vi "初始化.vi"(3 "Container State":T8 caption="容器状态", 4 "Previous State":variant caption="前期状态", 5 "Previous Version":T7 caption="前期版本") -> (2 "Current State":T1 caption="当前状态" {"配置信息"."间隔启动"."启动命令" items=["", "水样测试", "标样核查", "零点核查", "跨度核查", "空白测试", "平行样测试", "加标回收", "空白校准", "标样校准"]; "配置信息"."定点周期"."启动命令 24" items=["", "水样测试", "标样核查", "零点核查", "跨度核查", "空白测试", "平行样测试", "加标回收", "空白校准", "标样校准"]; "配置信息"."定点周期"."启动命令 23" items=["", "水样测试", "标样核查", "零点核查", "跨度核查", "空白测试", "平行样测试", "加标回收", "空白校准", "标样校准"]; "配置信息"."定点周期"."启动命令 22" items=["", "水样测试", "标样核查", "零点核查", "跨度核查", "空白测试", "平行样测试", "加标回收", "空白校准", "标样校准"]; "配置信息"."定点周期"."启动命令 21" items=["", "水样测试", "标样核查", "零点核查", "跨度核查", "空白测试", "平行样测试", "加标回收", "空白校准", "标样校准"]; "配置信息"."定点周期"."启动命令 20" items=["", "水样测试", "标样核查", "零点核查", "跨度核查", "空白测试", "平行样测试", "加标回收", "空白校准", "标样校准"]; "配置信息"."定点周期"."启动命令 19" items=["", "水样测试", "标样核查", "零点核查", "跨度核查", "空白测试", "平行样测试", "加标回收", "空白校准", "标样校准"]; "配置信息"."定点周期"."启动命令 18" items=["", "水样测试", "标样核查", "零点核查", "跨度核查", "空白测试", "平行样测试", "加标回收", "空白校准", "标样校准"]; "配置信息"."定点周期"."启动命令 17" items=["", "水样测试", "标样核查", "零点核查", "跨度核查", "空白测试", "平行样测试", "加标回收", "空白校准", "标样校准"]; "配置信息"."定点周期"."启动命令 16" items=["", "水样测试", "标样核查", "零点核查", "跨度核查", "空白测试", "平行样测试", "加标回收", "空白校准", "标样校准"]; "配置信息"."定点周期"."启动命令 15" items=["", "水样测试", "标样核查", "零点核查", "跨度核查", "空白测试", "平行样测试", "加标回收", "空白校准", "标样校准"]; "配置信息"."定点周期"."启动命令 14" items=["", "水样测试", "标样核查", "零点核查", "跨度核查", "空白测试", "平行样测试", "加标回收", "空白校准", "标样校准"]; "配置信息"."定点周期"."启动命令 13" items=["", "水样测试", "标样核查", "零点核查", "跨度核查", "空白测试", "平行样测试", "加标回收", "空白校准", "标样校准"]; "配置信息"."定点周期"."启动命令 12" items=["", "水样测试", "标样核查", "零点核查", "跨度核查", "空白测试", "平行样测试", "加标回收", "空白校准", "标样校准"]; "配置信息"."定点周期"."启动命令 11" items=["", "水样测试", "标样核查", "零点核查", "跨度核查", "空白测试", "平行样测试", "加标回收", "空白校准", "标样校准"]; "配置信息"."定点周期"."启动命令 10" items=["", "水样测试", "标样核查", "零点核查", "跨度核查", "空白测试", "平行样测试", "加标回收", "空白校准", "标样校准"]; "配置信息"."定点周期"."启动命令 9" items=["", "水样测试", "标样核查", "零点核查", "跨度核查", "空白测试", "平行样测试", "加标回收", "空白校准", "标样校准"]; "配置信息"."定点周期"."启动命令 8" items=["", "水样测试", "标样核查", "零点核查", "跨度核查", "空白测试", "平行样测试", "加标回收", "空白校准", "标样校准"]; "配置信息"."定点周期"."启动命令 7" items=["", "水样测试", "标样核查", "零点核查", "跨度核查", "空白测试", "平行样测试", "加标回收", "空白校准", "标样校准"]; "配置信息"."定点周期"."启动命令 6" items=["", "水样测试", "标样核查", "零点核查", "跨度核查", "空白测试", "平行样测试", "加标回收", "空白校准", "标样校准"]; "配置信息"."定点周期"."启动命令 5" items=["", "水样测试", "标样核查", "零点核查", "跨度核查", "空白测试", "平行样测试", "加标回收", "空白校准", "标样校准"]; "配置信息"."定点周期"."启动命令 4" items=["", "水样测试", "标样核查", "零点核查", "跨度核查", "空白测试", "平行样测试", "加标回收", "空白校准", "标样校准"]; "配置信息"."定点周期"."启动命令 3" items=["", "水样测试", "标样核查", "零点核查", "跨度核查", "空白测试", "平行样测试", "加标回收", "空白校准", "标样校准"]; "配置信息"."定点周期"."启动命令 2" items=["", "水样测试", "标样核查", "零点核查", "跨度核查", "空白测试", "平行样测试", "加标回收", "空白校准", "标样校准"]; "配置信息"."定点周期"."启动命令" items=["", "水样测试", "标样核查", "零点核查", "跨度核查", "空白测试", "平行样测试", "加标回收", "空白校准", "标样校准"]})   [LabVIEW 2016, in "定时设置.xctl"]
uses:
  <vilib>/_xctls/Container State.ctl
  <vilib>/_xctls/Version.ctl
  <vilib>/_xctls/XControlSupport.lvlib
panel:
  in  "Default Indicator State":T1 caption="默认显示控件状态" {"配置信息"."间隔启动"."启动命令" items=["", "水样测试", "标样核查", "零点核查", "跨度核查", "空白测试", "平行样测试", "加标回收", "空白校准", "标样校准"]; "配置信息"."定点周期"."启动命令 24" items=["", "水样测试", "标样核查", "零点核查", "跨度核查", "空白测试", "平行样测试", "加标回收", "空白校准", "标样校准"]; "配置信息"."定点周期"."启动命令 23" items=["", "水样测试", "标样核查", "零点核查", "跨度核查", "空白测试", "平行样测试", "加标回收", "空白校准", "标样校准"]; "配置信息"."定点周期"."启动命令 22" items=["", "水样测试", "标样核查", "零点核查", "跨度核查", "空白测试", "平行样测试", "加标回收", "空白校准", "标样校准"]; "配置信息"."定点周期"."启动命令 21" items=["", "水样测试", "标样核查", "零点核查", "跨度核查", "空白测试", "平行样测试", "加标回收", "空白校准", "标样校准"]; "配置信息"."定点周期"."启动命令 20" items=["", "水样测试", "标样核查", "零点核查", "跨度核查", "空白测试", "平行样测试", "加标回收", "空白校准", "标样校准"]; "配置信息"."定点周期"."启动命令 19" items=["", "水样测试", "标样核查", "零点核查", "跨度核查", "空白测试", "平行样测试", "加标回收", "空白校准", "标样校准"]; "配置信息"."定点周期"."启动命令 18" items=["", "水样测试", "标样核查", "零点核查", "跨度核查", "空白测试", "平行样测试", "加标回收", "空白校准", "标样校准"]; "配置信息"."定点周期"."启动命令 17" items=["", "水样测试", "标样核查", "零点核查", "跨度核查", "空白测试", "平行样测试", "加标回收", "空白校准", "标样校准"]; "配置信息"."定点周期"."启动命令 16" items=["", "水样测试", "标样核查", "零点核查", "跨度核查", "空白测试", "平行样测试", "加标回收", "空白校准", "标样校准"]; "配置信息"."定点周期"."启动命令 15" items=["", "水样测试", "标样核查", "零点核查", "跨度核查", "空白测试", "平行样测试", "加标回收", "空白校准", "标样校准"]; "配置信息"."定点周期"."启动命令 14" items=["", "水样测试", "标样核查", "零点核查", "跨度核查", "空白测试", "平行样测试", "加标回收", "空白校准", "标样校准"]; "配置信息"."定点周期"."启动命令 13" items=["", "水样测试", "标样核查", "零点核查", "跨度核查", "空白测试", "平行样测试", "加标回收", "空白校准", "标样校准"]; "配置信息"."定点周期"."启动命令 12" items=["", "水样测试", "标样核查", "零点核查", "跨度核查", "空白测试", "平行样测试", "加标回收", "空白校准", "标样校准"]; "配置信息"."定点周期"."启动命令 11" items=["", "水样测试", "标样核查", "零点核查", "跨度核查", "空白测试", "平行样测试", "加标回收", "空白校准", "标样校准"]; "配置信息"."定点周期"."启动命令 10" items=["", "水样测试", "标样核查", "零点核查", "跨度核查", "空白测试", "平行样测试", "加标回收", "空白校准", "标样校准"]; "配置信息"."定点周期"."启动命令 9" items=["", "水样测试", "标样核查", "零点核查", "跨度核查", "空白测试", "平行样测试", "加标回收", "空白校准", "标样校准"]; "配置信息"."定点周期"."启动命令 8" items=["", "水样测试", "标样核查", "零点核查", "跨度核查", "空白测试", "平行样测试", "加标回收", "空白校准", "标样校准"]; "配置信息"."定点周期"."启动命令 7" items=["", "水样测试", "标样核查", "零点核查", "跨度核查", "空白测试", "平行样测试", "加标回收", "空白校准", "标样校准"]; "配置信息"."定点周期"."启动命令 6" items=["", "水样测试", "标样核查", "零点核查", "跨度核查", "空白测试", "平行样测试", "加标回收", "空白校准", "标样校准"]; "配置信息"."定点周期"."启动命令 5" items=["", "水样测试", "标样核查", "零点核查", "跨度核查", "空白测试", "平行样测试", "加标回收", "空白校准", "标样校准"]; "配置信息"."定点周期"."启动命令 4" items=["", "水样测试", "标样核查", "零点核查", "跨度核查", "空白测试", "平行样测试", "加标回收", "空白校准", "标样校准"]; "配置信息"."定点周期"."启动命令 3" items=["", "水样测试", "标样核查", "零点核查", "跨度核查", "空白测试", "平行样测试", "加标回收", "空白校准", "标样校准"]; "配置信息"."定点周期"."启动命令 2" items=["", "水样测试", "标样核查", "零点核查", "跨度核查", "空白测试", "平行样测试", "加标回收", "空白校准", "标样校准"]; "配置信息"."定点周期"."启动命令" items=["", "水样测试", "标样核查", "零点核查", "跨度核查", "空白测试", "平行样测试", "加标回收", "空白校准", "标样校准"]}
  in  "Default Control State":T1 caption="默认输入控件状态" {"配置信息"."间隔启动"."启动命令" items=["", "水样测试", "标样核查", "零点核查", "跨度核查", "空白测试", "平行样测试", "加标回收", "空白校准", "标样校准"]; "配置信息"."定点周期"."启动命令 24" items=["", "水样测试", "标样核查", "零点核查", "跨度核查", "空白测试", "平行样测试", "加标回收", "空白校准", "标样校准"]; "配置信息"."定点周期"."启动命令 23" items=["", "水样测试", "标样核查", "零点核查", "跨度核查", "空白测试", "平行样测试", "加标回收", "空白校准", "标样校准"]; "配置信息"."定点周期"."启动命令 22" items=["", "水样测试", "标样核查", "零点核查", "跨度核查", "空白测试", "平行样测试", "加标回收", "空白校准", "标样校准"]; "配置信息"."定点周期"."启动命令 21" items=["", "水样测试", "标样核查", "零点核查", "跨度核查", "空白测试", "平行样测试", "加标回收", "空白校准", "标样校准"]; "配置信息"."定点周期"."启动命令 20" items=["", "水样测试", "标样核查", "零点核查", "跨度核查", "空白测试", "平行样测试", "加标回收", "空白校准", "标样校准"]; "配置信息"."定点周期"."启动命令 19" items=["", "水样测试", "标样核查", "零点核查", "跨度核查", "空白测试", "平行样测试", "加标回收", "空白校准", "标样校准"]; "配置信息"."定点周期"."启动命令 18" items=["", "水样测试", "标样核查", "零点核查", "跨度核查", "空白测试", "平行样测试", "加标回收", "空白校准", "标样校准"]; "配置信息"."定点周期"."启动命令 17" items=["", "水样测试", "标样核查", "零点核查", "跨度核查", "空白测试", "平行样测试", "加标回收", "空白校准", "标样校准"]; "配置信息"."定点周期"."启动命令 16" items=["", "水样测试", "标样核查", "零点核查", "跨度核查", "空白测试", "平行样测试", "加标回收", "空白校准", "标样校准"]; "配置信息"."定点周期"."启动命令 15" items=["", "水样测试", "标样核查", "零点核查", "跨度核查", "空白测试", "平行样测试", "加标回收", "空白校准", "标样校准"]; "配置信息"."定点周期"."启动命令 14" items=["", "水样测试", "标样核查", "零点核查", "跨度核查", "空白测试", "平行样测试", "加标回收", "空白校准", "标样校准"]; "配置信息"."定点周期"."启动命令 13" items=["", "水样测试", "标样核查", "零点核查", "跨度核查", "空白测试", "平行样测试", "加标回收", "空白校准", "标样校准"]; "配置信息"."定点周期"."启动命令 12" items=["", "水样测试", "标样核查", "零点核查", "跨度核查", "空白测试", "平行样测试", "加标回收", "空白校准", "标样校准"]; "配置信息"."定点周期"."启动命令 11" items=["", "水样测试", "标样核查", "零点核查", "跨度核查", "空白测试", "平行样测试", "加标回收", "空白校准", "标样校准"]; "配置信息"."定点周期"."启动命令 10" items=["", "水样测试", "标样核查", "零点核查", "跨度核查", "空白测试", "平行样测试", "加标回收", "空白校准", "标样校准"]; "配置信息"."定点周期"."启动命令 9" items=["", "水样测试", "标样核查", "零点核查", "跨度核查", "空白测试", "平行样测试", "加标回收", "空白校准", "标样校准"]; "配置信息"."定点周期"."启动命令 8" items=["", "水样测试", "标样核查", "零点核查", "跨度核查", "空白测试", "平行样测试", "加标回收", "空白校准", "标样校准"]; "配置信息"."定点周期"."启动命令 7" items=["", "水样测试", "标样核查", "零点核查", "跨度核查", "空白测试", "平行样测试", "加标回收", "空白校准", "标样校准"]; "配置信息"."定点周期"."启动命令 6" items=["", "水样测试", "标样核查", "零点核查", "跨度核查", "空白测试", "平行样测试", "加标回收", "空白校准", "标样校准"]; "配置信息"."定点周期"."启动命令 5" items=["", "水样测试", "标样核查", "零点核查", "跨度核查", "空白测试", "平行样测试", "加标回收", "空白校准", "标样校准"]; "配置信息"."定点周期"."启动命令 4" items=["", "水样测试", "标样核查", "零点核查", "跨度核查", "空白测试", "平行样测试", "加标回收", "空白校准", "标样校准"]; "配置信息"."定点周期"."启动命令 3" items=["", "水样测试", "标样核查", "零点核查", "跨度核查", "空白测试", "平行样测试", "加标回收", "空白校准", "标样校准"]; "配置信息"."定点周期"."启动命令 2" items=["", "水样测试", "标样核查", "零点核查", "跨度核查", "空白测试", "平行样测试", "加标回收", "空白校准", "标样校准"]; "配置信息"."定点周期"."启动命令" items=["", "水样测试", "标样核查", "零点核查", "跨度核查", "空白测试", "平行样测试", "加标回收", "空白校准", "标样校准"]}
  # "分钟"
  # "次"
  # "分钟"
  # "次"
  # "分钟"
  # "次"
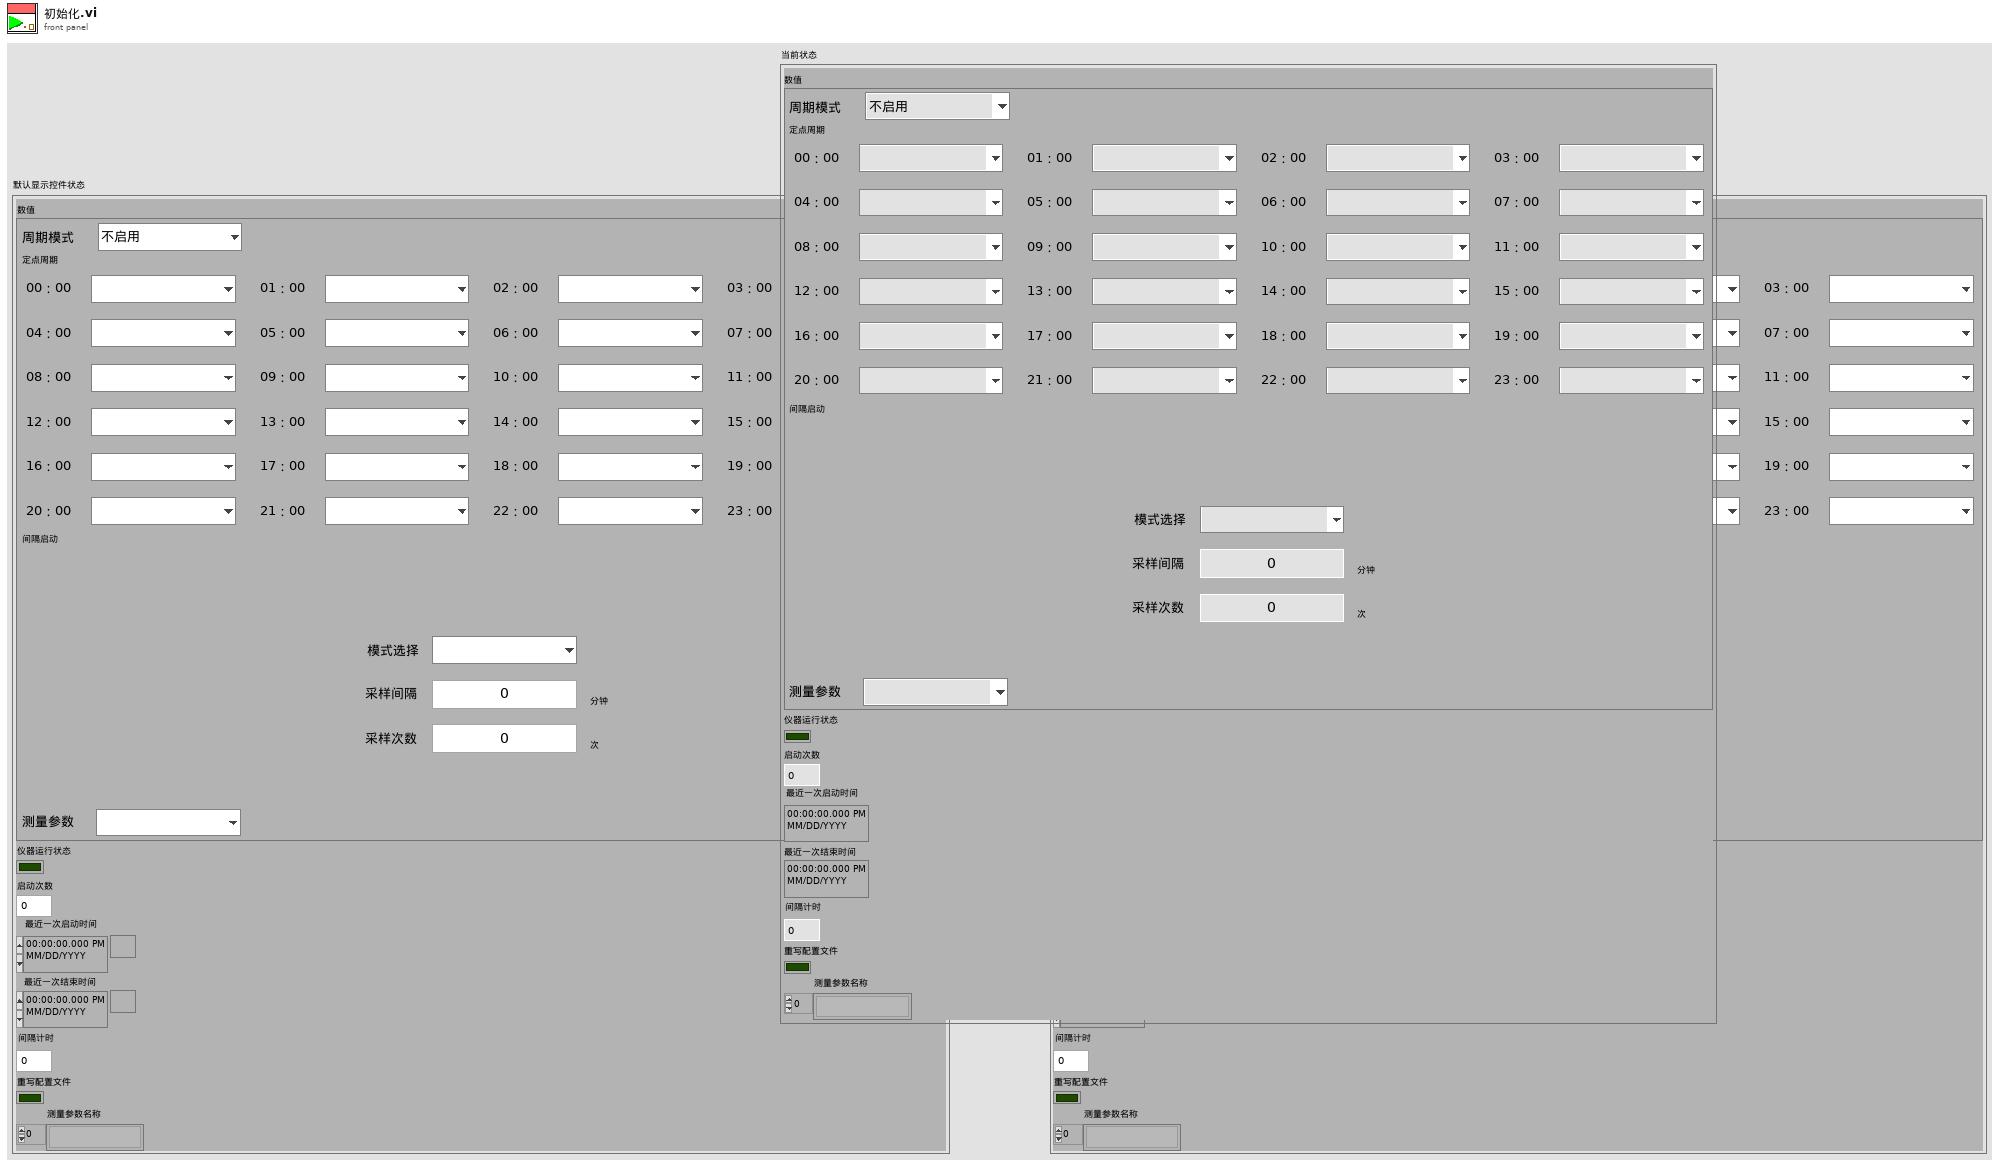
[diagram p1: front panel]
types:
  T1 = typedef "定时设置.xctl/状态.ctl" = cluster{"配置信息":cluster{"周期模式":T2, "定点周期":T3, "间隔启动":T5, "测量参数":T6}, "仪器运行状态":bool, "启动次数":i32, "最近一次启动时间":timestamp, "最近一次结束时间":timestamp, "间隔计时":dbl, "重写配置文件":bool, "测量参数名称":string[]}
  T2 = typedef "定时设置.xctl/周期模式设置.ctl" = enum16{"不启用", "定点模式", "间隔模式"}
  T3 = typedef "定时设置.xctl/定点周期设置.ctl" = cluster{"启动命令":T4, "启动命令 2":T4, "启动命令 3":T4, "启动命令 4":T4, "启动命令 5":T4, "启动命令 6":T4, "启动命令 7":T4, "启动命令 8":T4, "启动命令 9":T4, "启动命令 10":T4, "启动命令 11":T4, "启动命令 12":T4, "启动命令 13":T4, "启动命令 14":T4, "启动命令 15":T4, "启动命令 16":T4, "启动命令 17":T4, "启动命令 18":T4, "启动命令 19":T4, "启动命令 20":T4, "启动命令 21":T4, "启动命令 22":T4, "启动命令 23":T4, "启动命令 24":T4}
  T4 = typedef "定时设置.xctl/启动命令选择.ctl" = u16
  T5 = typedef "定时设置.xctl/间隔启动设置.ctl" = cluster{"启动命令":T4, "启动间隔":dbl, "启动次数":i32}
  T6 = typedef "定时设置.xctl/测量参数.ctl" = u16
  T7 = typedef "XControlSupport.lvlib/Version.ctl" = cluster{"Major":u16, "Minor":u16, "Fix":u16, "Build":u16}
  T8 = typedef "XControlSupport.lvlib/Container State.ctl" = cluster{"Indicator?":bool, "Run Mode?":bool, " Refnum":refnum<vi>}
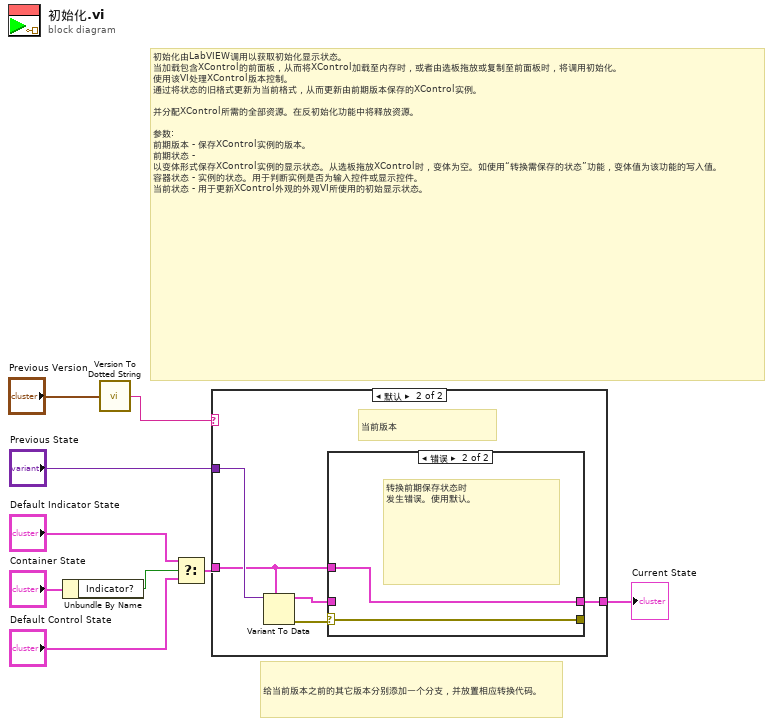
[diagram p0: block diagram]
diagram:
  # "给当前版本之前的其它版本分别添加一个分支，并放置相应转换代码。"
  # "初始化由LabVIEW调用以获取初始化显示状态。\n当加载包含XControl的前面板，从而将XControl加载至内存时，或者由选板拖放或复制至前面板时，将调用初始化。\n使用该VI处理XControl版本控制。\n通过将状态的旧格式更新为当前格式，从而更新由前期版本保存的XControl实例。\n\n并分配XControl所需的全部资源。在反初始化功能中将释放资源。\n\n参数: \n前期版本 - 保存XControl实例的版本。\n前期状态 - 以变体形式保存XControl实例的显示状态。从选板拖放XControl时，变体为空。如使用“转换需保存的状态”功能，变体值为该功能的写入值。\n容器状态 - 实例的状态。用于判断实例是否为输入控件或显示控件。\n当前状态 - 用于更新XControl外观的外观VI所使用的初始显示状态。"
  n1 = Unbundle By Name("Container State") -> ("Indicator?"=w4:bool)
  n2 = call <vilib>:"Version To Dotted String.vi"("Version"="Previous Version") -> ("String Version"=w1:string)
  n3 = Select(t="Default Indicator State", s=w4, f="Default Control State") -> (s? t:f=w3:T1)
  n4 = case shown="默认" w1 {
    tunnel: "Previous State" -> [_ w15]
    tunnel: [w10 w11] -> w8
    tunnel: w3 -> [w10 w12]
    frame "0.0.0.0" {
      # "已创建，并使用默认状态"
    }
    frame Default {
      # "当前版本"
      n5 = Variant To Data(type=w12, Variant=w15) -> (data=w13:T1, error out=w14:errorcluster)  [unwired: 1 in]
      n6 = case shown="错误" w14 {
        selector: w14 -> [w17 w18]
        tunnel: w13 -> [w16 _]
        tunnel: [w16 w19] -> w11
        tunnel: w12 -> [_ w19]
        tunnel: [w17 w18] -> _
        frame No Error {
        }
        frame Error {
          # "转换前期保存状态时\n发生错误。使用默认。"
        }
      }
    }
  }
  "Current State" <- w8
